vi "Manipulator Controller.vi"   [LabVIEW 2018]
uses:
  <vilib>/Rock Robotics/WPI/Joystick/WPI_JoystickDeviceEnum.ctl
  Manipulator Controller Global.vi
types:
  T1 = typedef "WPI_JoystickDeviceEnum.ctl" = enum16{"USB 0", "USB 1", "USB 2", "USB 3", "USB 4", "USB 5"}
  T2 = typedef "WPI_JoystickDevRef.ctl" = cluster{"Device":T1}
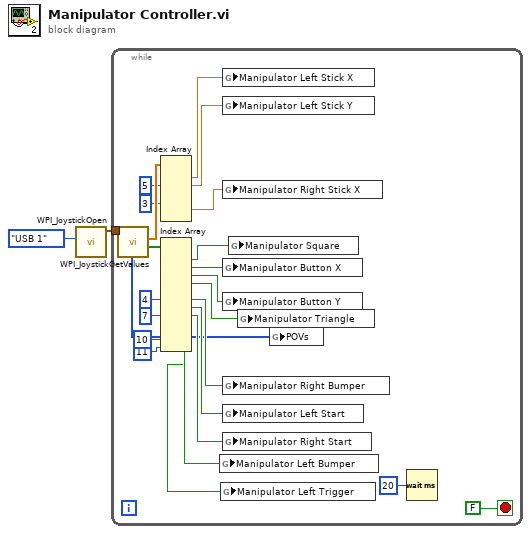
[diagram p0: block diagram]
diagram:
  n1 = call <vilib>:"WPI_JoystickOpen.vi"("JoystickDevice"=WPI_JoystickDeviceEnum."USB 1") -> ("JoystickDevRef"=w1:T2)  [unwired: 10 in]
  n2 = while {
    tunnel: w1 -> [w26]
    stop <- FALSE stop-if-true
    n3 = call <vilib>:"WPI_JoystickGetValues.vi"("JoystickDevRef"=w26) -> ("Buttons"=w24:bool[], "Axes"=w25:dbl[], "POVs"=w8:i16[])  [unwired: 6 in, 2 out]
    n4 = Index Array(array=w25, index #2=5 ("index"), index #4=3 ("index")) -> (element #1=w23:dbl, element #2=w22:dbl, element #5=w21:dbl)  [unwired: 4 in, 3 out]
    n5 = Index Array(array=w24, index #6=4 ("index"), index #8=7 ("index"), index #11=10 ("index"), index #12=11 ("index")) -> (element #1=w20:bool, element #2=w19:bool, element #3=w18:bool, element #4=w7:bool, element #6=w17:bool, element #7=w16:bool, element #8=w15:bool, element #11=w5:bool, element #12=w3:bool)  [unwired: 8 in, 3 out]
    n6 = global write "Manipulator Controller Global.vi" "Manipulator Left Bumper"(w5) -> ()
    n7 = global write "Manipulator Controller Global.vi" "Manipulator Left Trigger"(w3) -> ()
    n8 = global write "Manipulator Controller Global.vi" "Manipulator Left Stick X"(w23) -> ()
    n9 = global write "Manipulator Controller Global.vi" "Manipulator Left Stick Y"(w22) -> ()
    n10 = global write "Manipulator Controller Global.vi" "Manipulator Right Stick X"(w21) -> ()
    n11 = global write "Manipulator Controller Global.vi" "Manipulator Button X"(w19) -> ()
    n12 = global write "Manipulator Controller Global.vi" "Manipulator Button Y"(w18) -> ()
    n13 = global write "Manipulator Controller Global.vi" "Manipulator Right Bumper"(w17) -> ()
    n14 = global write "Manipulator Controller Global.vi" "Manipulator Left Start"(w16) -> ()
    n15 = global write "Manipulator Controller Global.vi" "Manipulator Right Start"(w15) -> ()
    n16 = global write "Manipulator Controller Global.vi" "Manipulator Square"(w20) -> ()
    n17 = global write "Manipulator Controller Global.vi" "Manipulator Triangle"(w7) -> ()
    n18 = global write "Manipulator Controller Global.vi" "POVs"(w8) -> ()
    n19 = Wait (ms)(milliseconds to wait=u32 20) -> ()  [unwired: 1 out]
  }
